vi "get voltage range ring.vi"(8 "error in (no error)":errorcluster caption="에러 입력(에러 없음)", 11 "Haptic IC 입력":refnum<class "Haptic IC.lvclass">) -> (0 "error out":errorcluster caption="에러 출력", 1 "caption":string, 2 "strings & values":T1, 3 "Haptic IC 출력":refnum<class "Haptic IC.lvclass">, 4 "read value":dbl)   [LabVIEW 2020, in "Haptic IC.lvclass"]
uses:
  Haptic IC.lvclass
  <vilib>/Utility/miscctls.llb/LVStringsAndValuesArrayTypeDef_DBL.ctl
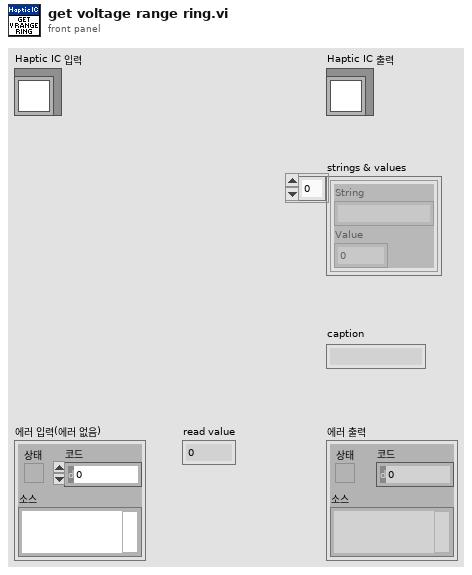
[diagram p1: front panel]
types:
  T1 = typedef "LVStringsAndValuesArrayTypeDef_DBL.ctl" = cluster{"String":string, "Value":dbl}[]
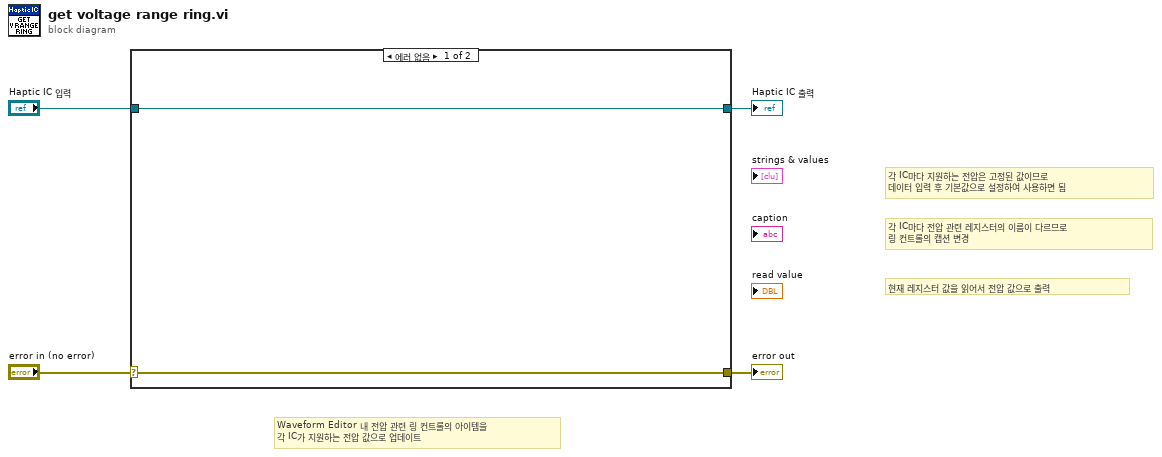
[diagram p0: block diagram]
diagram:
  # "현재 레지스터 값을 읽어서 전압 값으로 출력"
  # "각 IC마다 전압 관련 레지스터의 이름이 다르므로\n링 컨트롤의 캡션 변경"
  # "각 IC마다 지원하는 전압은 고정된 값이므로\n데이터 입력 후 기본값으로 설정하여 사용하면 됨"
  # "Waveform Editor 내 전압 관련 링 컨트롤의 아이템을\n각 IC가 지원하는 전압 값으로 업데이트"
  n1 = case shown="에러 없음" "error in (no error)" {
    selector: "error in (no error)" -> [w5 w8]
    tunnel: [w5 w8] -> w3
    tunnel: [w6 w7] -> w1
    tunnel: "Haptic IC 입력" -> [w6 w7]
    frame No Error {
    }
    frame Error {
    }
  }
  "error out" <- w3
  "Haptic IC 출력" <- w1
